vi "Add Debug Line.vi"(10 "Debug Line":string, 11 "Engine in":refnum<class "Engine.lvclass">) -> ()   [LabVIEW 2020, in "TSnax.lvlib" / "Engine.lvclass"]
uses:
  Engine.lvclass
  Engine.lvclass/Engine.ctl
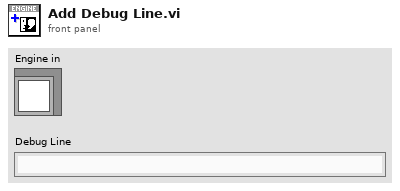
[diagram p1: front panel]
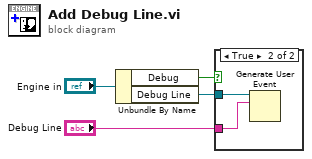
[diagram p0: block diagram]
diagram:
  n1 = Unbundle By Name("Engine in") -> ("Debug"=w3:bool, "Debug Line"=w2:refnum<user-event>)
  n2 = case shown="True" w3 {
    tunnel: w2 -> [_ w6]
    tunnel: "Debug Line" -> [_ w5]
    frame False {
    }
    frame True {
      n3 = Generate User Event(user event=w6, event data cluster=w5) -> ()  [unwired: 2 in, 2 out]
    }
  }
